vi "Delete User.vi"(8 "error in (no error)":errorcluster, 10 "Credential":T1, 11 "MySQL in":refnum<class "MySQL.lvclass">) -> (0 "error out":errorcluster, 3 "MySQL out":refnum<class "MySQL.lvclass">)   [LabVIEW 2021, in "Database.lvlib" / "MySQL.lvclass"]
uses:
  MySQL.lvclass
  DB/Credential.ctl
  DB/DB.lvclass
  Database.lvlib
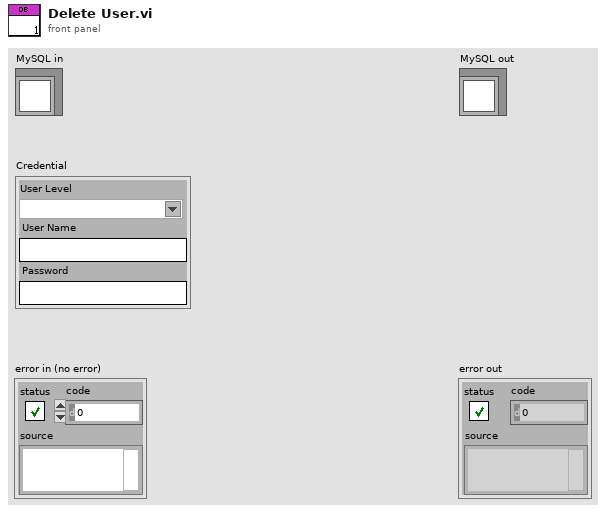
[diagram p1: front panel]
types:
  T1 = typedef "Database.lvlib/Credential.ctl" = cluster{"User Level":string, "User Name":string, "Password":string}
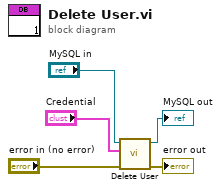
[diagram p0: block diagram]
diagram:
  n1 = call-parent "Delete User.vi"("error in (no error)"="error in (no error)", "Credential"="Credential", "DB in"="MySQL in") -> ("error out"=→"error out":errorcluster, "DB out"=→"MySQL out":refnum<class "MySQL.lvclass">)  [unwired: 7 in]
